vi "Convert from Celcius to fahrenhit.vi"() -> ()   [LabVIEW 2022 SP3]
panel:
  out "Tf":dbl
  in  "Tc":dbl
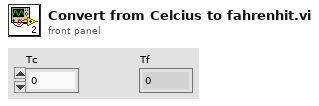
[diagram p1: front panel]
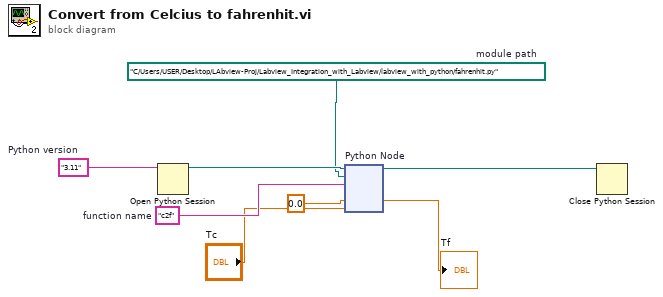
[diagram p0: block diagram]
diagram:
  w5 = "c2f"  # function name
  w6 = path "C:/Users/USER/Desktop/LAbview-Proj/Labview_Integration_with_Labview/labview_with_python/fahrenhit.py"  # module path
  w8 = "3.11"  # Python version
  n1 = Open Python Session(python version=w8) -> (session out=w7:refnum<k35>)  [unwired: 2 in, 1 out]
  n2 = node "Python Node"(w7, w6, w5, 0.0, "Tc") -> (w1:refnum<k35>, →"Tf":dbl)  [unwired: 2 in, 3 out]
  n3 = Close Python Session(session in=w1) -> ()  [unwired: 1 in, 1 out]
